vi "programar_con_jlink.vi"() -> ()   [LabVIEW 2023]
uses:
  controls/Exit button.ctl
  <vilib>/Utility/sysdir.llb/System Directory Type.ctl
panel:
  in  "Tab Control":enum32{"Programm", "Configuration"}(tab)
  in  "Blank Button":bool
  in  "Play Button":bool
  in  "Select .mot file":path
  out "Output":string
  in  "PASSWORD":string(combo)
  in  "select device":string(combo)="R5F52317"
  in  "speed":string(combo)="1000"
  in  "Connection type":string(combo)="FINE"
  in  "Action":enum16{"Erase", "Erase and upload", "Upload"}(ring)=enum."Erase and upload"
  in  "Stop Button":T1
  # "Aún no funciona el RL78"
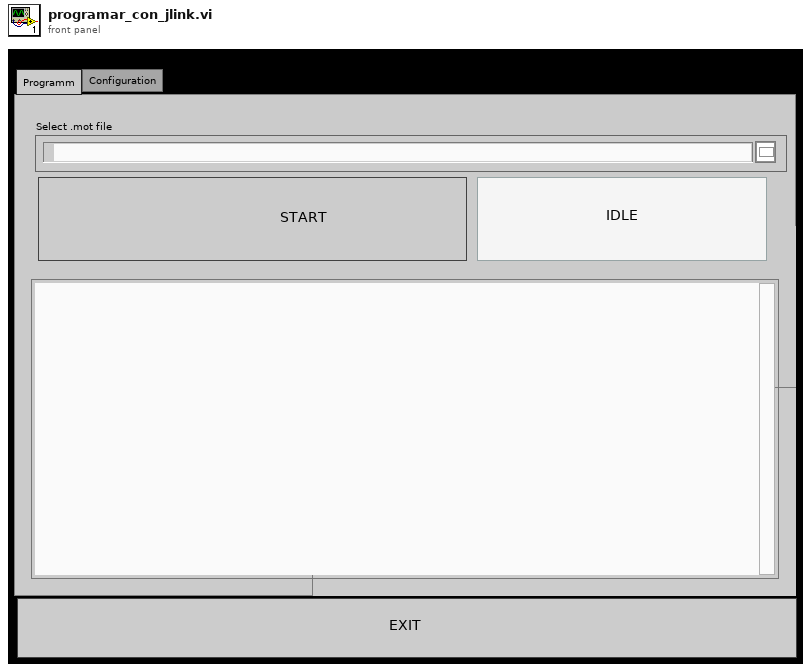
[diagram p1: front panel]
types:
  T1 = typedef "Exit button.ctl" = bool
  T2 = typedef "System Directory Type.ctl" = i32
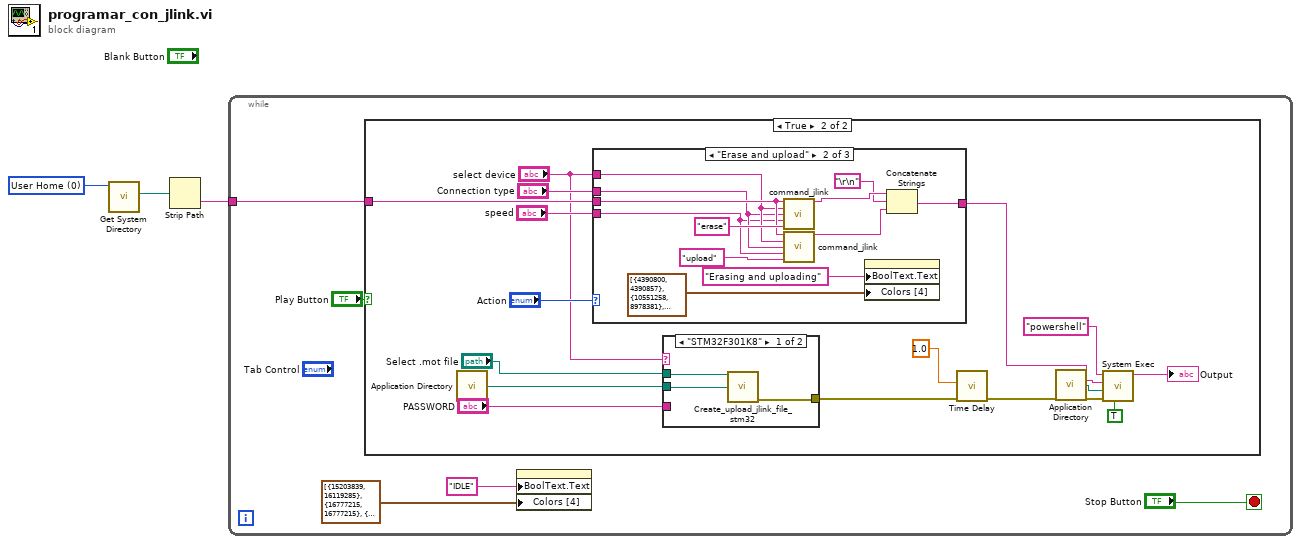
[diagram p0: block diagram]
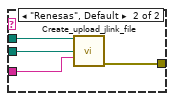
[diagram p3: hidden frame]
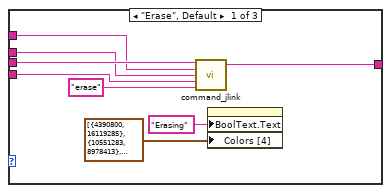
[diagram p4: hidden frame]
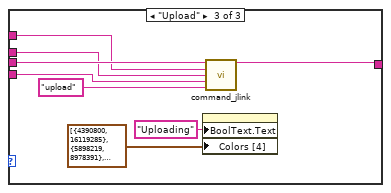
[diagram p5: hidden frame]
diagram:
  w2 = T2 0 items=["User Home"=0, "User Desktop"=1, "User Documents"=2, "User Application Data"=3, "User Preferences"=4, "User Temporary"=5, "Public Documents"=6, "Public Application Data"=7, "Public Preferences"=8, "Public Cache"=13, "System Core Libraries"=9, "System Installed Libraries"=10, "Application Files"=11, "Boot Volume Root"=12] ("system directory type")
  n1 = call <vilib>:"Get System Directory.vi"("system directory type"=w2) -> ("system directory"=w3:path)  [unwired: 10 in]
  n2 = Strip Path(path=w3) -> (name=w1:string)  [unwired: 1 out]
  n3 = while {
    tunnel: w1 -> [w4]
    stop <- "Stop Button" stop-if-true
    n4 = case shown="True" "Play Button" {
      tunnel: w4 -> [_ w14]
      frame False {
      }
      frame True {
        n5 = call <vilib>:"Application Directory.vi"() -> ("Application Directory"=w17:path)
        n6 = case shown="\"Erase and upload\"" "Action" {
          tunnel: w14 -> [w37 w48 w57]
          tunnel: "select device" -> [w36 w47 w56]
          tunnel: "Connection type" -> [w35 w46 w55]
          tunnel: "speed" -> [w34 w45 w54]
          tunnel: [w32 w43 w52] -> w11
          frame "Erase", Default {
            n7 = call "command_jlink.vi"("user"=w37, "Device"=w36, "conection type"=w35, "speed"=w34, "uploader_erase?"="erase") -> ("command_jlink"=w32:string)  [unwired: 10 in]
            n8 = property on="Blank Button" class="Bool"("BoolText.Text"="Erasing" ("Boolean Text.Text"), "Colors [4]"=cluster{u32, u32}[] [{4390800, 16119285}, {10551283, 8978413}, {10551283, 10551283}, {65511, 16770137}]) -> ()  [unwired: 2 in, 2 out]
          }
          frame "Erase and upload" {
            n9 = call "command_jlink.vi"("user"=w48, "Device"=w47, "conection type"=w46, "speed"=w45, "uploader_erase?"="erase") -> ("command_jlink"=w42:string)  [unwired: 10 in]
            n10 = call "command_jlink.vi"("user"=w48, "Device"=w47, "conection type"=w46, "speed"=w45, "uploader_erase?"="upload") -> ("command_jlink"=w40:string)  [unwired: 10 in]
            n11 = property on="Blank Button" class="Bool"("BoolText.Text"="Erasing and uploading" ("Boolean Text.Text"), "Colors [4]"=cluster{u32, u32}[] [{4390800, 4390857}, {10551258, 8978381}, {10551283, 10551283}, {65511, 16770137}]) -> ()  [unwired: 2 in, 2 out]
            n12 = Concatenate Strings(w42, "\r\n", w40) -> (w43:string)
          }
          frame "Upload" {
            n13 = property on="Blank Button" class="Bool"("BoolText.Text"="Uploading" ("Boolean Text.Text"), "Colors [4]"=cluster{u32, u32}[] [{4390800, 16119285}, {5898219, 8978391}, {10551283, 10551283}, {65511, 16770137}]) -> ()  [unwired: 2 in, 2 out]
            n14 = call "command_jlink.vi"("user"=w57, "Device"=w56, "conection type"=w55, "speed"=w54, "uploader_erase?"="upload") -> ("command_jlink"=w52:string)  [unwired: 10 in]
          }
        }
        n15 = case shown="\"STM32F301K8\"" "select device" {
          tunnel: [w27 w31] -> w19
          tunnel: "Select .mot file" -> [w26 w30]
          tunnel: w17 -> [w25 w29]
          tunnel: "PASSWORD" -> [_ w28]
          frame "STM32F301K8" {
            n16 = call "Create_upload_jlink_file_stm32.vi"(".mot file"=w26, "path"=w25) -> ("error out"=w27:errorcluster)  [unwired: 13 in]
          }
          frame "Renesas", Default {
            n17 = call "Create_upload_jlink_file.vi"(".mot file"=w30, "path"=w29, "Password"=w28) -> ("error out"=w31:errorcluster)  [unwired: 12 in]
          }
        }
        n18 = call "Time Delay"("error in (no error)"=w19, "Delay Time (s)"=1.0) -> ("error out"=w23:errorcluster)  [unwired: 9 in]
        n19 = call <vilib>:"Application Directory.vi"() -> ("Application Directory"=w21:path)
        n20 = call <vilib>:"System Exec.vi"("run minimized? (F)"=TRUE, "error in (no error)"=w23, "working directory"=w21, "standard input"=w11, "command line"="powershell") -> ("standard output"=→"Output":string)  [unwired: 3 in, 3 out]
      }
    }
    n21 = property on="Blank Button" class="Bool"("BoolText.Text"="IDLE" ("Boolean Text.Text"), "Colors [4]"=cluster{u32, u32}[] [{15203839, 16119285}, {16777215, 16777215}, {0, 0}, {65511, 16770137}]) -> ()  [unwired: 2 in, 2 out]
  }
